vi "Auto Drive XY Center Switch.vi"(0 "RobotDriveDevRef In":T2={"DevStatus"={"status"=FALSE, "code"=0, "source"=""}, "Motors[]"=[], "Square Inputs"=FALSE, "Max Output"=1.0}, 1 "Angle Offset":dbl, 3 "Movement":dbl=-1.0, 5 "Motor Output Range X":cluster{"output high":dbl, "output low":dbl}={"output high"=0.8, "output low"=-0.8}, 7 "PID Gains X":T1={"proportional gain (Kc)"=0.07, "integral time (Ti, min)"=0.0, "derivative time (Td, min)"=0.0}, 9 "Distance (in)":dbl=15.0 format="%#_13g", 11 "Time to Settle (ms)":u32=50, 12 "Min Time (ms)":u32=250, 13 "PID Gains Y":T1={"proportional gain (Kc)"=0.07, "integral time (Ti, min)"=0.0, "derivative time (Td, min)"=0.0}, 14 "Motor Output Range Y":cluster{"output high":dbl, "output low":dbl}={"output high"=0.7, "output low"=-0.7}, 15 "Max Time (ms)":u32=15000) -> (4 "RobotDriveDevRef Out":T2={"DevStatus"={"status"=FALSE, "code"=0, "source"=""}, "Motors[]"=[], "Square Inputs"=FALSE, "Max Output"=1.0})   [LabVIEW 2017]
uses:
  <vilib>/Rock Robotics/WPI/RobotDrive/WPI_RobotDriveDevRef.ctl
  <vilib>/Rock Robotics/WPI/MotorControl/WPI_MotorControlDeviceRef.ctl
  <vilib>/Rock Robotics/WPI/MotorControl/WPI_MotorControlType.ctl
  <vilib>/Rock Robotics/SystemInterfaces/DIO/FPGA_DIOPWMChannel.ctl
  <vilib>/Rock Robotics/WPI/PWM/WPI_PWMDeadband.ctl
  <vilib>/Rock Robotics/SystemInterfaces/DIO/FPGA_DIOChannel.ctl
  <vilib>/Rock Robotics/WPI/Solenoid/WPI_SolenoidValue.ctl
  Globals/Robot Global Data.vi
  <vilib>/addons/control/pid/pid.llb/PID (DBL).vi
  <vilib>/Rock Robotics/WPI/RobotDrive/WPI_RobotDriveArcadeDrive_Standard(NoSaturation).vi
  <vilib>/addons/control/pid/NI_PID_pid.lvlib
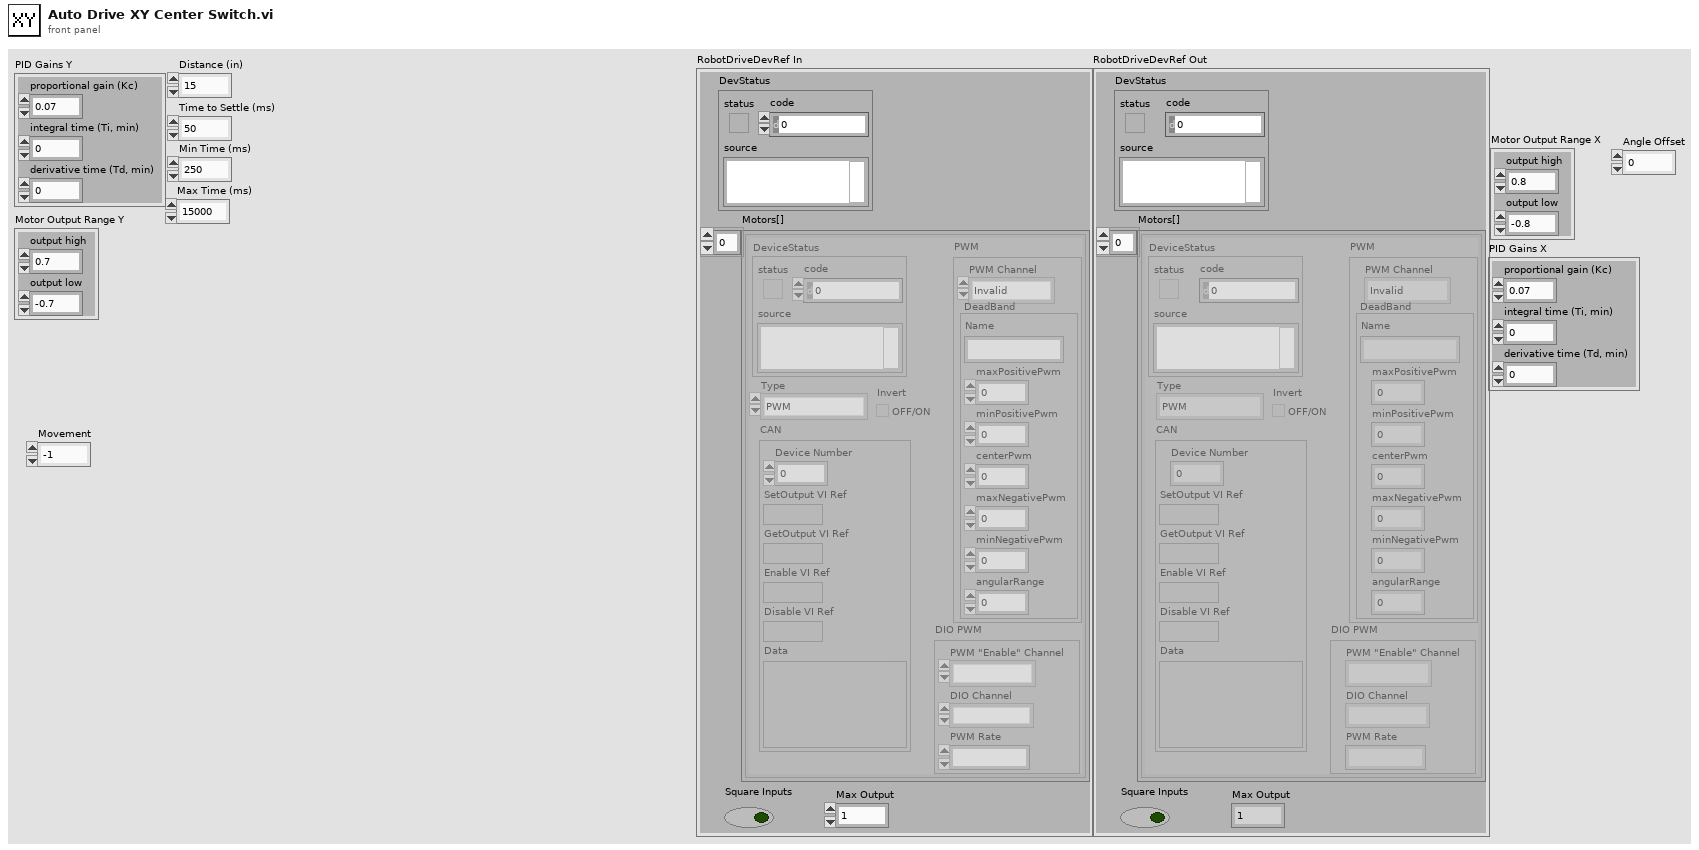
[diagram p1: front panel]
types:
  T1 = cluster{"proportional gain (Kc)":dbl, "integral time (Ti, min)":dbl, "derivative time (Td, min)":dbl}
  T2 = typedef "WPI_RobotDriveDevRef.ctl" = cluster{"DevStatus":errorcluster, "Motors[]":T3[], "Square Inputs":bool, "Max Output":dbl}
  T3 = typedef "WPI_MotorControlDeviceRef.ctl" = cluster{"DeviceStatus":errorcluster, "Type":T4, "PWM":cluster{"PWM Channel":T5, "DeadBand":T6}, "CAN":cluster{"Device Number":u8, "SetOutput VI Ref":variant, "GetOutput VI Ref":variant, "Enable VI Ref":variant, "Disable VI Ref":variant, "Data":variant}, "Invert":bool, "DIO PWM":cluster{"PWM \"Enable\" Channel":T5, "DIOChannel":T7, "PWM Rate":dbl}}
  T4 = typedef "WPI_MotorControlType.ctl" = enum16{"PWM", "CAN", "DIO PWM"}
  T5 = typedef "FPGA_DIOPWMChannel.ctl" = enum8{"PWM 0", "PWM 1", "PWM 2", "PWM 3", "PWM 4", "PWM 5", "PWM 6", "PWM 7", "PWM 8", "PWM 9", "PWM MXP 0", "PWM MXP 1", "PWM MXP 2", "PWM MXP 3", "PWM MXP 4", "PWM MXP 5", "PWM MXP 6", "PWM MXP 7", "PWM MXP 8", "PWM MXP 9", "Invalid"}
  T6 = typedef "WPI_PWMDeadband.ctl" = cluster{"Name":string, "maxPositivePwm":i32, "minPositivePwm":i32, "centerPwm":i32, "maxNegativePwm":i32, "minNegativePwm":i32, "angularRange":u16}
  T7 = typedef "FPGA_DIOChannel.ctl" = enum8{"DIO 0", "DIO 1", "DIO 2", "DIO 3", "DIO 4", "DIO 5", "DIO 6", "DIO 7", "DIO 8", "DIO 9", "DIO MXP 0", "DIO MXP 1", "DIO MXP 2", "DIO MXP 3", "DIO MXP 4", "DIO MXP 5", "DIO MXP 6", "DIO MXP 7", "DIO MXP 8", "DIO MXP 9", "DIO MXP 10", "DIO MXP 11", "DIO MXP 12", "DIO MXP 13", "DIO MXP 14", "DIO MXP 15", "SPI Port CS1", "SPI Port CS2", "SPI Port CS3", "SPI Port MISO", "SPI Port MOSI", "Invalid"}
  T8 = typedef "WPI_SolenoidValue.ctl" = enum16{"Off", "On", "Forward", "Reverse"}
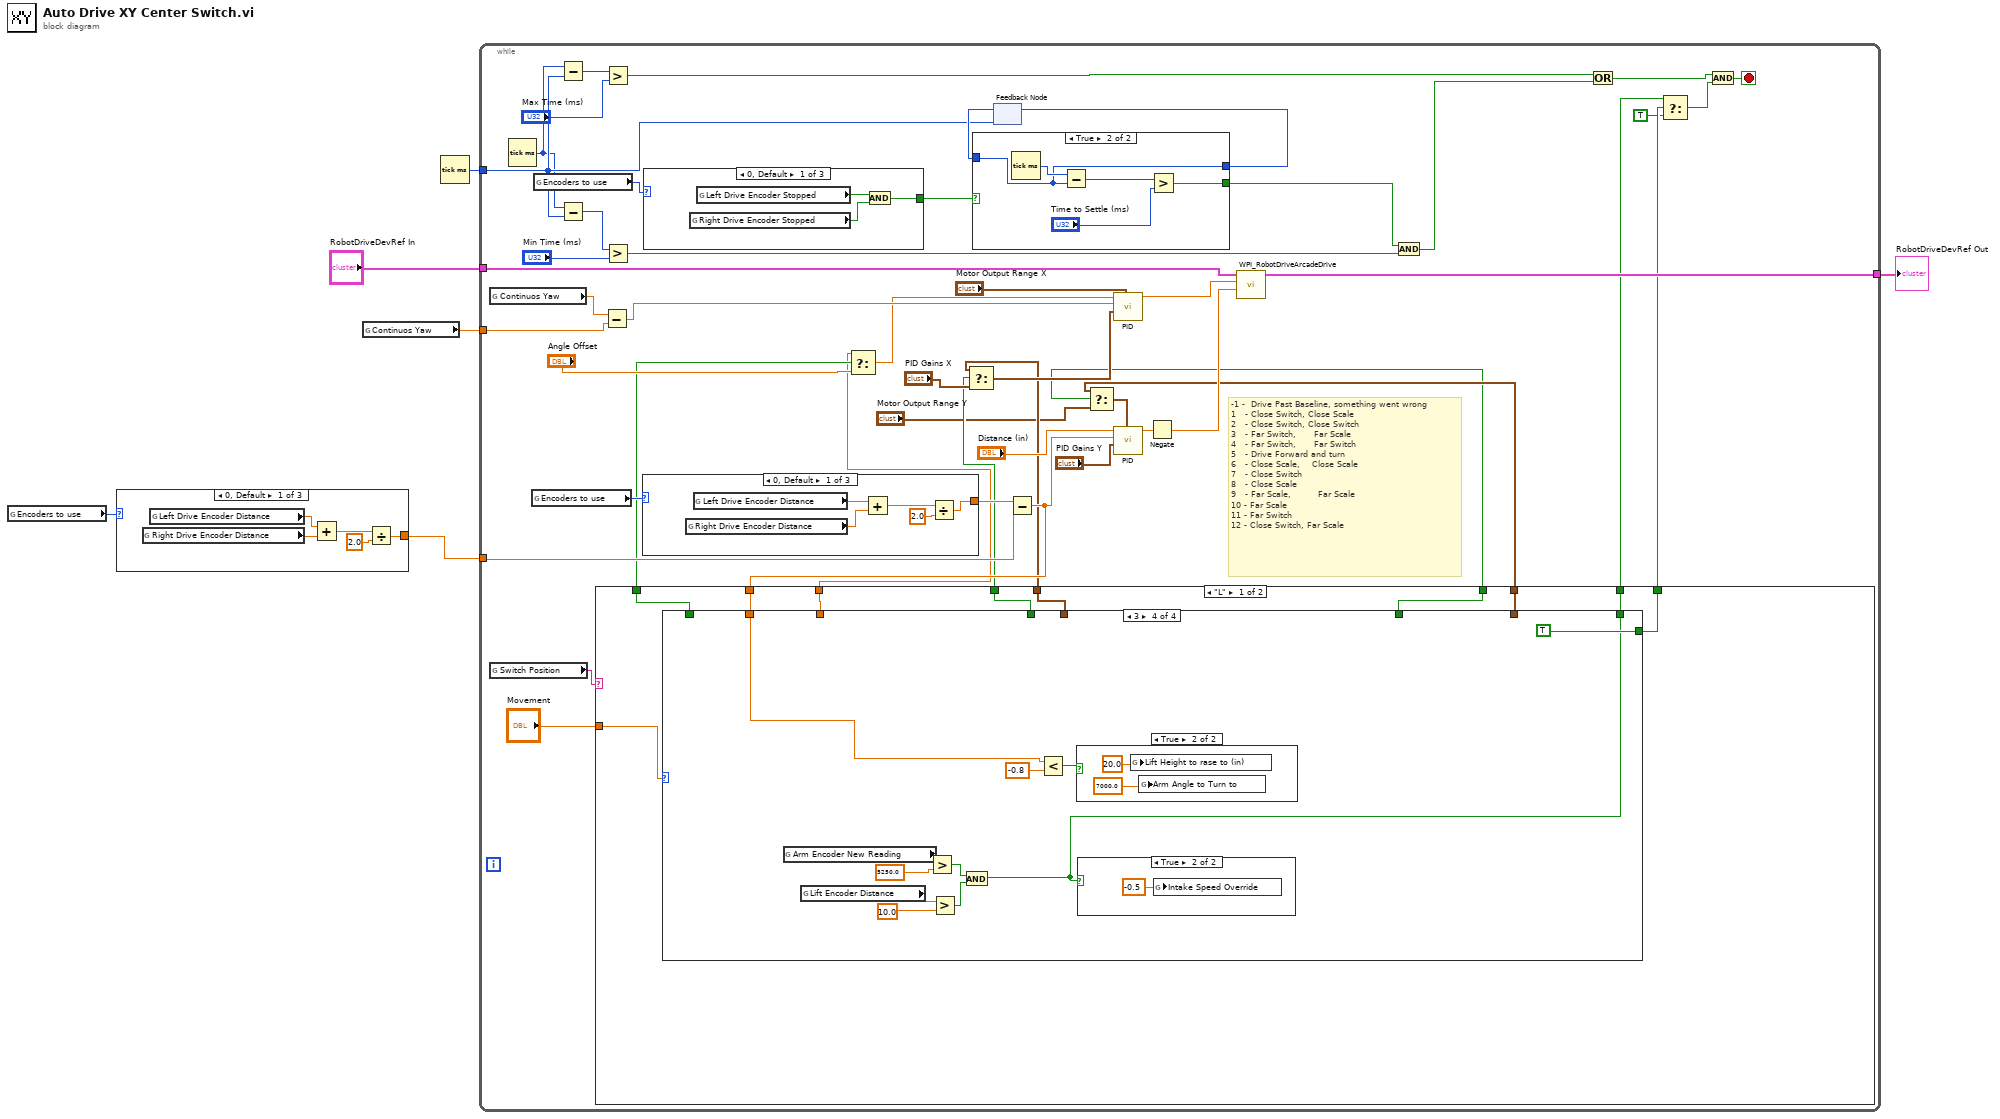
[diagram p0: block diagram]
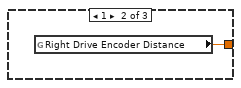
[diagram p2: hidden frame]
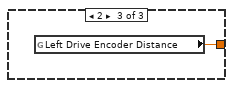
[diagram p3: hidden frame]
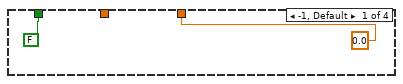
[diagram p4: hidden frame]
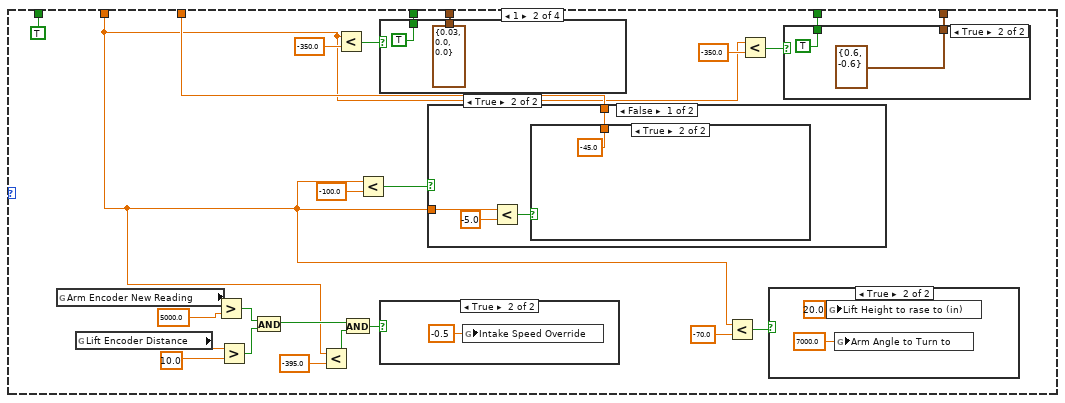
[diagram p5: hidden frame]
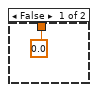
[diagram p10: hidden frame]
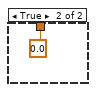
[diagram p11: hidden frame]
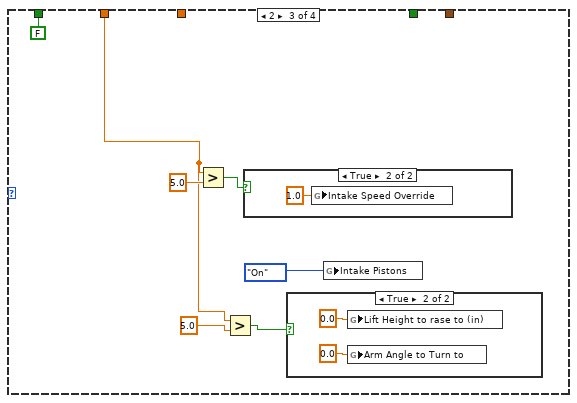
[diagram p12: hidden frame]
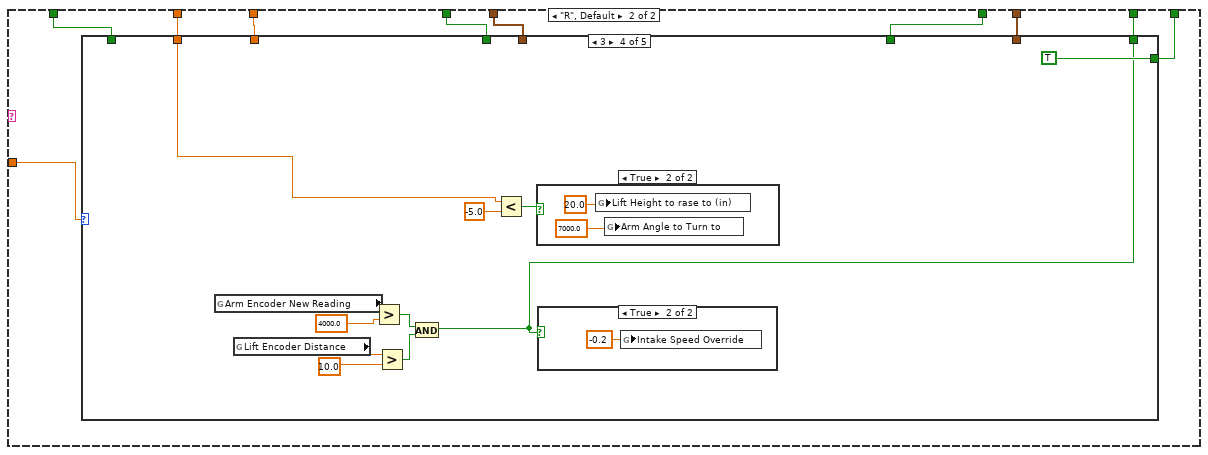
[diagram p17: hidden frame]
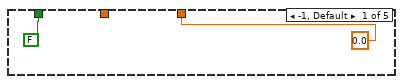
[diagram p18: hidden frame]
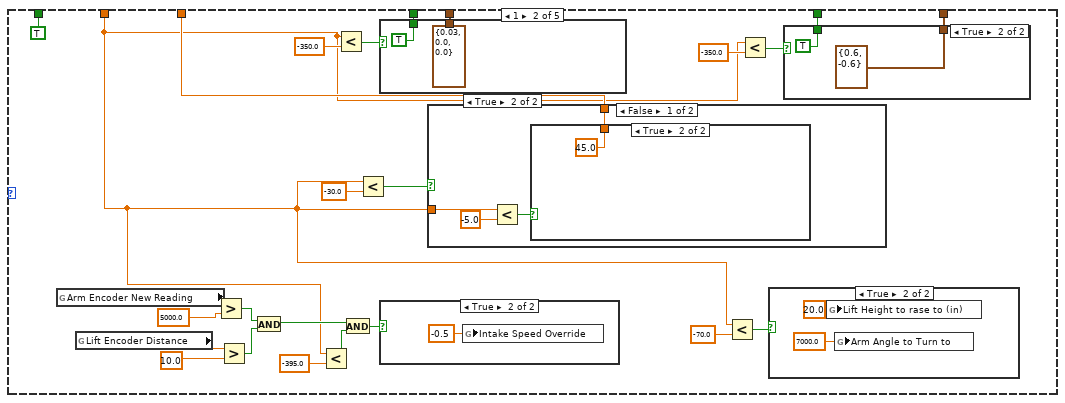
[diagram p19: hidden frame]
diagram:
  n1 = global read "Robot Global Data.vi" "Encoders to use"() -> (w2:u16)
  n2 = case shown="0, Default" w2 {
    tunnel: [w7 w12 w13] -> w6
    frame 0, Default {
      n3 = global read "Robot Global Data.vi" "Right Drive Encoder Distance"() -> (w10:dbl)
      n4 = global read "Robot Global Data.vi" "Left Drive Encoder Distance"() -> (w11:dbl)
      n5 = Add(x=w11, y=w10) -> (x+y=w9:dbl)
      n6 = Divide(x=w9, y=2.0) -> (x/y=w7:dbl)
    }
    frame 1 {
      n7 = global read "Robot Global Data.vi" "Right Drive Encoder Distance"() -> (w12:dbl)
    }
    frame 2 {
      n8 = global read "Robot Global Data.vi" "Left Drive Encoder Distance"() -> (w13:dbl)
    }
  }
  n9 = global read "Robot Global Data.vi" "Continuos Yaw"() -> (w1:dbl)
  n10 = Tick Count (ms)() -> (millisecond timer value=w5:u32)
  n11 = while {
    tunnel: "RobotDriveDevRef In" -> [w60]
    tunnel: w6 -> [w55]
    tunnel: w5 -> [w45]
    tunnel: [w54] -> w4
    tunnel: w1 -> [w36]
    stop <- w19 stop-if-true
    # "-1 -  Drive Past Baseline, something went wrong\n1   - Close Switch, Close Scale\n2   - Close Switch, Close Switch\n3   - Far Switch,      Far Scale\n4   - Far Switch,      Far Switch\n5   - Drive Forward and turn\n6   - Close Scale,    Close Scale\n7   - Close Switch\n8   - Close Scale\n9   - Far Scale,         Far Scale\n10 - Far Scale\n11 - Far Switch\n12 - Close Switch, Far Scale"
    n12 = global read "Robot Global Data.vi" "Continuos Yaw"() -> (w37:dbl)
    n13 = global read "Robot Global Data.vi" "Switch Position"() -> (w29:string)
    n14 = Tick Count (ms)() -> (millisecond timer value=w44:u32)
    n15 = global read "Robot Global Data.vi" "Encoders to use"() -> (w43:u16)
    n16 = global read "Robot Global Data.vi" "Encoders to use"() -> (w41:u16)
    n17 = Subtract(x=w44, y=w45) -> (x-y=w48:u32)
    n18 = Subtract(x=w44, y=w45) -> (x-y=w53:u32)
    n19 = Subtract(x=w37, y=w36) -> (x-y=w35:dbl)
    n20 = Greater?(x=w48, y="Max Time (ms)") -> (0:w46:bool)
    n21 = Greater?(x=w53, y="Min Time (ms)") -> (0:w50:bool)
    n22 = case shown="0, Default" w43 {
      tunnel: [w239 w244 w245] -> w42
      frame 0, Default {
        n23 = global read "Robot Global Data.vi" "Right Drive Encoder Distance"() -> (w242:dbl)
        n24 = global read "Robot Global Data.vi" "Left Drive Encoder Distance"() -> (w243:dbl)
        n25 = Add(x=w243, y=w242) -> (x+y=w241:dbl)
        n26 = Divide(x=w241, y=2.0) -> (x/y=w239:dbl)
      }
      frame 1 {
        n27 = global read "Robot Global Data.vi" "Right Drive Encoder Distance"() -> (w244:dbl)
      }
      frame 2 {
        n28 = global read "Robot Global Data.vi" "Left Drive Encoder Distance"() -> (w245:dbl)
      }
    }
    n29 = case shown="0, Default" w41 {
      tunnel: [w236 w237 w238] -> w40
      frame 0, Default {
        n30 = global read "Robot Global Data.vi" "Right Drive Encoder Stopped"() -> (w234:bool)
        n31 = global read "Robot Global Data.vi" "Left Drive Encoder Stopped"() -> (w235:bool)
        n32 = And(x=w235, y=w234) -> (x .and. y?=w236:bool)
      }
      frame 1 {
        n33 = global read "Robot Global Data.vi" "Right Drive Encoder Stopped"() -> (w237:bool)
      }
      frame 2 {
        n34 = global read "Robot Global Data.vi" "Left Drive Encoder Stopped"() -> (w238:bool)
      }
    }
    n35 = feedback #1(w45) -> (w56:u32)
    n36 = case shown="True" w40 {
      tunnel: w56 -> [_ w251]
      tunnel: [w247 w251] -> w57
      tunnel: [FALSE w248] -> w51
      frame False {
        n37 = Tick Count (ms)() -> (millisecond timer value=w247:u32)
      }
      frame True {
        n38 = Tick Count (ms)() -> (millisecond timer value=w252:u32)
        n39 = Subtract(x=w252, y=w251) -> (x-y=w250:u32)
        n40 = Greater?(x=w250, y="Time to Settle (ms)") -> (0:w248:bool)
      }
    }
    n41 = feedback-in #1(w57) -> ()
    n42 = Subtract(x=w42, y=w55) -> (x-y=w33:dbl)
    n43 = case shown="\"L\"" w29 {
      tunnel: "Movement" -> [w72 w147]
      tunnel: w33 -> [w69 w144]
      tunnel: [w71 w146] -> w30
      tunnel: [w70 w145] -> w28
      tunnel: [w67 w142] -> w25
      tunnel: [w68 w143] -> w24
      tunnel: [w65 w140] -> w21
      tunnel: [w66 w141] -> w20
      tunnel: [w64 w139] -> w16
      tunnel: [w63 w138] -> w15
      frame "L" {
        n44 = case shown="3" w72 {
          tunnel: [FALSE TRUE FALSE _] -> w71
          tunnel: [0.0 w98 _ _] -> w70
          tunnel: w69 -> [_ w76 w114 w126]
          tunnel: [_ w93 _ _] -> w68
          tunnel: [_ w92 _ _] -> w67
          tunnel: [_ w77 _ _] -> w66
          tunnel: [_ w75 _ _] -> w65
          tunnel: [_ _ _ TRUE] -> w64
          tunnel: [_ _ _ w124] -> w63
          frame -1, Default {
          }
          frame 1 {
            n45 = global read "Robot Global Data.vi" "Arm Encoder New Reading"() -> (w90:dbl)
            n46 = global read "Robot Global Data.vi" "Lift Encoder Distance"() -> (w91:dbl)
            n47 = Greater?(x=w90, y=5000.0 ("Arm Angle to Turn to")) -> (0:w87:bool)
            n48 = Greater?(x=w91, y=10.0 ("Arm Angle to Turn to")) -> (0:w86:bool)
            n49 = And(x=w87, y=w86) -> (x .and. y?=w82:bool)
            n50 = Less?(x=w76, y=-395.0) -> (x < y?=w83:bool)
            n51 = Less?(x=w76, y=-350.0) -> (x < y?=w94:bool)
            n52 = And(x=w82, y=w83) -> (x .and. y?=w84:bool)
            n53 = Less?(x=w76, y=-100.0) -> (x < y?=w96:bool)
            n54 = case shown="True" w94 {
              tunnel: [_ T1 {"proportional gain (Kc)"=0.03, "integral time (Ti, min)"=0.0, "derivative time (Td, min)"=0.0} ("t")] -> w93
              tunnel: [_ TRUE] -> w92
              frame False {
              }
              frame True {
              }
            }
            n55 = case shown="True" w84 {
              frame False {
              }
              frame True {
                n56 = global write "Robot Global Data.vi" "Intake Speed Override"(-0.5 ("Arm Angle to Turn to")) -> ()
              }
            }
            n57 = case shown="False" w96 {
              tunnel: [w108 0.0] -> w98
              tunnel: w76 -> [w107 _]
              frame False {
                n58 = Less?(x=w107, y=-5.0) -> (x < y?=w110:bool)
                n59 = case shown="True" w110 {
                  tunnel: [0.0 -45.0] -> w108
                  frame False {
                  }
                  frame True {
                  }
                }
              }
              frame True {
              }
            }
            n60 = Less?(x=w76, y=-70.0) -> (x < y?=w80:bool)
            n61 = Less?(x=w76, y=-350.0) -> (x < y?=w78:bool)
            n62 = case shown="True" w80 {
              frame False {
              }
              frame True {
                n63 = global write "Robot Global Data.vi" "Lift Height to rase to (in)"(20.0 ("Arm Angle to Turn to")) -> ()
                n64 = global write "Robot Global Data.vi" "Arm Angle to Turn to"(7000.0 ("Arm Angle to Turn to")) -> ()
              }
            }
            n65 = case shown="True" w78 {
              tunnel: [_ TRUE] -> w77
              tunnel: [_ cluster{"output high":dbl, "output low":dbl} {"output high"=0.6, "output low"=-0.6} ("s? t:f")] -> w75
              frame False {
              }
              frame True {
              }
            }
          }
          frame 2 {
            n66 = Greater?(x=w114, y=5.0) -> (0:w118:bool)
            n67 = Greater?(x=w114, y=5.0) -> (0:w116:bool)
            n68 = case shown="True" w118 {
              frame False {
              }
              frame True {
                n69 = global write "Robot Global Data.vi" "Intake Speed Override"(1.0 ("Arm Angle to Turn to")) -> ()
              }
            }
            n70 = case shown="True" w116 {
              frame False {
              }
              frame True {
                n71 = global write "Robot Global Data.vi" "Lift Height to rase to (in)"(0.0 ("Arm Angle to Turn to")) -> ()
                n72 = global write "Robot Global Data.vi" "Arm Angle to Turn to"(0.0 ("Arm Angle to Turn to")) -> ()
              }
            }
            n73 = global write "Robot Global Data.vi" "Intake Pistons"(WPI_SolenoidValue."On" ("Intake Pistons")) -> ()
          }
          frame 3 {
            n74 = global read "Robot Global Data.vi" "Arm Encoder New Reading"() -> (w133:dbl)
            n75 = global read "Robot Global Data.vi" "Lift Encoder Distance"() -> (w134:dbl)
            n76 = Greater?(x=w133, y=5250.0 ("Arm Angle to Turn to")) -> (0:w130:bool)
            n77 = Greater?(x=w134, y=10.0 ("Arm Angle to Turn to")) -> (0:w129:bool)
            n78 = And(x=w130, y=w129) -> (x .and. y?=w124:bool)
            n79 = Less?(x=w126, y=-0.8) -> (x < y?=w127:bool)
            n80 = case shown="True" w127 {
              frame False {
              }
              frame True {
                n81 = global write "Robot Global Data.vi" "Lift Height to rase to (in)"(20.0 ("Lift Height to rase to (in)")) -> ()
                n82 = global write "Robot Global Data.vi" "Arm Angle to Turn to"(7000.0 ("Lift Height to rase to (in)")) -> ()
              }
            }
            n83 = case shown="True" w124 {
              frame False {
              }
              frame True {
                n84 = global write "Robot Global Data.vi" "Intake Speed Override"(-0.5 ("Arm Angle to Turn to")) -> ()
              }
            }
          }
        }
      }
      frame "R", Default {
        n85 = case shown="3" w147 {
          tunnel: [FALSE TRUE FALSE _ _] -> w146
          tunnel: [0.0 w173 _ _ w213] -> w145
          tunnel: w144 -> [_ w151 w189 w201 w214]
          tunnel: [_ w168 _ _ _] -> w143
          tunnel: [_ w167 _ _ _] -> w142
          tunnel: [_ w152 _ _ _] -> w141
          tunnel: [_ w150 _ _ _] -> w140
          tunnel: [_ _ _ TRUE _] -> w139
          tunnel: [_ _ _ w199 w215] -> w138
          frame -1, Default {
          }
          frame 1 {
            n86 = global read "Robot Global Data.vi" "Arm Encoder New Reading"() -> (w165:dbl)
            n87 = global read "Robot Global Data.vi" "Lift Encoder Distance"() -> (w166:dbl)
            n88 = Greater?(x=w165, y=5000.0 ("Arm Angle to Turn to")) -> (0:w162:bool)
            n89 = Greater?(x=w166, y=10.0 ("Arm Angle to Turn to")) -> (0:w161:bool)
            n90 = And(x=w162, y=w161) -> (x .and. y?=w157:bool)
            n91 = Less?(x=w151, y=-395.0) -> (x < y?=w158:bool)
            n92 = Less?(x=w151, y=-350.0) -> (x < y?=w169:bool)
            n93 = And(x=w157, y=w158) -> (x .and. y?=w159:bool)
            n94 = Less?(x=w151, y=-30.0) -> (x < y?=w171:bool)
            n95 = case shown="True" w169 {
              tunnel: [_ T1 {"proportional gain (Kc)"=0.03, "integral time (Ti, min)"=0.0, "derivative time (Td, min)"=0.0} ("t")] -> w168
              tunnel: [_ TRUE] -> w167
              frame False {
              }
              frame True {
              }
            }
            n96 = case shown="True" w159 {
              frame False {
              }
              frame True {
                n97 = global write "Robot Global Data.vi" "Intake Speed Override"(-0.5 ("Arm Angle to Turn to")) -> ()
              }
            }
            n98 = case shown="False" w171 {
              tunnel: [w183 0.0] -> w173
              tunnel: w151 -> [w182 _]
              frame False {
                n99 = Less?(x=w182, y=-5.0) -> (x < y?=w185:bool)
                n100 = case shown="True" w185 {
                  tunnel: [0.0 45.0] -> w183
                  frame False {
                  }
                  frame True {
                  }
                }
              }
              frame True {
              }
            }
            n101 = Less?(x=w151, y=-70.0) -> (x < y?=w155:bool)
            n102 = Less?(x=w151, y=-350.0) -> (x < y?=w153:bool)
            n103 = case shown="True" w155 {
              frame False {
              }
              frame True {
                n104 = global write "Robot Global Data.vi" "Lift Height to rase to (in)"(20.0 ("Arm Angle to Turn to")) -> ()
                n105 = global write "Robot Global Data.vi" "Arm Angle to Turn to"(7000.0 ("Arm Angle to Turn to")) -> ()
              }
            }
            n106 = case shown="True" w153 {
              tunnel: [_ TRUE] -> w152
              tunnel: [_ cluster{"output high":dbl, "output low":dbl} {"output high"=0.6, "output low"=-0.6} ("s? t:f")] -> w150
              frame False {
              }
              frame True {
              }
            }
          }
          frame 2 {
            n107 = Greater?(x=w189, y=5.0) -> (0:w193:bool)
            n108 = Greater?(x=w189, y=5.0) -> (0:w191:bool)
            n109 = case shown="True" w193 {
              frame False {
              }
              frame True {
                n110 = global write "Robot Global Data.vi" "Intake Speed Override"(1.0 ("Arm Angle to Turn to")) -> ()
              }
            }
            n111 = case shown="True" w191 {
              frame False {
              }
              frame True {
                n112 = global write "Robot Global Data.vi" "Lift Height to rase to (in)"(0.0 ("Arm Angle to Turn to")) -> ()
                n113 = global write "Robot Global Data.vi" "Arm Angle to Turn to"(0.0 ("Arm Angle to Turn to")) -> ()
              }
            }
            n114 = global write "Robot Global Data.vi" "Intake Pistons"(WPI_SolenoidValue."On" ("Intake Pistons")) -> ()
          }
          frame 3 {
            n115 = global read "Robot Global Data.vi" "Arm Encoder New Reading"() -> (w208:dbl)
            n116 = global read "Robot Global Data.vi" "Lift Encoder Distance"() -> (w209:dbl)
            n117 = Greater?(x=w208, y=4000.0 ("Arm Angle to Turn to")) -> (0:w205:bool)
            n118 = Greater?(x=w209, y=10.0 ("Arm Angle to Turn to")) -> (0:w204:bool)
            n119 = And(x=w205, y=w204) -> (x .and. y?=w199:bool)
            n120 = Less?(x=w201, y=-5.0) -> (x < y?=w202:bool)
            n121 = case shown="True" w202 {
              frame False {
              }
              frame True {
                n122 = global write "Robot Global Data.vi" "Lift Height to rase to (in)"(20.0 ("Lift Height to rase to (in)")) -> ()
                n123 = global write "Robot Global Data.vi" "Arm Angle to Turn to"(7000.0 ("Lift Height to rase to (in)")) -> ()
              }
            }
            n124 = case shown="True" w199 {
              frame False {
              }
              frame True {
                n125 = global write "Robot Global Data.vi" "Intake Speed Override"(-0.2 ("Arm Angle to Turn to")) -> ()
              }
            }
          }
          frame 4 {
            n126 = disable-structure shown="Disabled" {
              disable-tunnel: [w220 _] -> w215
              disable-tunnel: w214 -> [w217 _]
              disable-tunnel: [w216 _] -> w213
              frame Disabled {
                n127 = global read "Robot Global Data.vi" "Arm Encoder New Reading"() -> (w227:dbl)
                n128 = global read "Robot Global Data.vi" "Lift Encoder Distance"() -> (w228:dbl)
                n129 = Less?(x=w217, y=-10.0) -> (x < y?=w218:bool)
                n130 = Greater?(x=w227, y=4000.0 ("Arm Angle to Turn to")) -> (0:w224:bool)
                n131 = Greater?(x=w228, y=10.0 ("Arm Angle to Turn to")) -> (0:w223:bool)
                n132 = case shown="True" w218 {
                  tunnel: [0.0 -115.0] -> w216
                  frame False {
                  }
                  frame True {
                  }
                }
                n133 = And(x=w224, y=w223) -> (x .and. y?=w220:bool)
                n134 = Less?(x=w217, y=-30.0) -> (x < y?=w221:bool)
                n135 = case shown="True" w221 {
                  frame False {
                  }
                  frame True {
                    n136 = global write "Robot Global Data.vi" "Lift Height to rase to (in)"(20.0 ("Lift Height to rase to (in)")) -> ()
                    n137 = global write "Robot Global Data.vi" "Arm Angle to Turn to"(7000.0 ("Lift Height to rase to (in)")) -> ()
                  }
                }
                n138 = case shown="True" w220 {
                  frame False {
                  }
                  frame True {
                    n139 = global write "Robot Global Data.vi" "Intake Speed Override"(-0.2 ("Arm Angle to Turn to")) -> ()
                  }
                }
              }
              frame Enabled {
              }
            }
          }
        }
      }
    }
    n140 = Select(t=w28, s=w30, f="Angle Offset") -> (s? t:f=w32:dbl)
    n141 = Select(t=w24, s=w25, f="PID Gains X") -> (s? t:f=w26:T1)
    n142 = Select(t=w21, s=w20, f="Motor Output Range Y") -> (s? t:f=w22:cluster{"output high":dbl, "output low":dbl})
    n143 = call-poly <vilib>:"PID.vi"("output range"="Motor Output Range X", "PID gains"=w26, "process variable"=w35, "setpoint"=w32) -> ("output"=w39:dbl)  [unwired: 6 in, 1 out]
    n144 = call-poly <vilib>:"PID.vi"("output range"=w22, "PID gains"="PID Gains Y", "process variable"=w33, "setpoint"="Distance (in)") -> ("output"=w58:dbl)  [unwired: 6 in, 1 out]
    n145 = Negate(x=w58) -> (-x=w59:dbl)
    n146 = call-poly <vilib>:"WPI_RobotDriveArcadeDrive.vi"("Y axis value"=w59, "X axis value"=w39, "RobotDriveDevRef"=w60) -> ("RobotDriveDevRef"=w54:T2)  [unwired: 6 in, 2 out]
    n147 = And(x=w51, y=w50) -> (x .and. y?=w47:bool)
    n148 = Or(x=w46, y=w47) -> (x .or. y?=w18:bool)
    n149 = Select(t=w15, s=w16, f=TRUE) -> (s? t:f=w17:bool)
    n150 = And(x=w18, y=w17) -> (x .and. y?=w19:bool)
  }
  "RobotDriveDevRef Out" <- w4
